vi "COMI WFM Start.vi"(5 "nMaxLoops":i32, 6 "nPPS":u32, 7 "nNumData":u32, 9 "pDataBuffer":sgl, 10 "ch":i32, 11 "hDevice":u32) -> (1 "pDataBuffer out":sgl, 2 "function return":i32, 3 "hDevice out":u32)   [LabVIEW 2017, in "Comidll.lvlib"]
doc: "long (COMI_WFM_Start) (HANDLE hDevice, int ch, float *pDataBuffer, \n unsigned int nNumData, unsigned int nPPS, int nMaxLoops);"
uses:
  <userlib>/Comidll/Comidll.lvlib
  <userlib>/Comidll/Comidll.dll
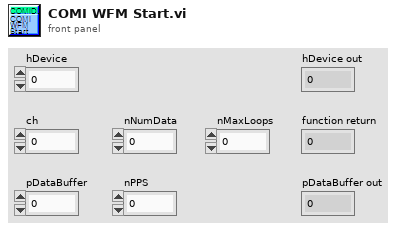
[diagram p1: front panel]
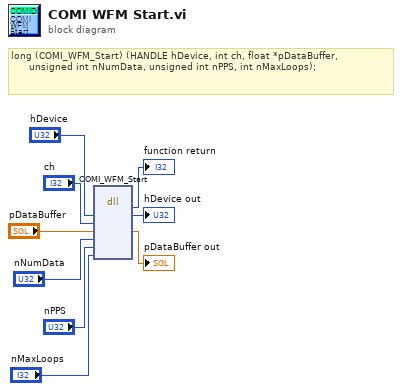
[diagram p0: block diagram]
diagram:
  # "long\t(COMI_WFM_Start) (HANDLE hDevice, int ch, float *pDataBuffer, \n\t\t\t\t\t\tunsigned int nNumData, unsigned int nPPS, int nMaxLoops);"
  n1 = dll-call lib="C:/Program Files/National Instruments/LabVIEW 2017/user.lib/Comidll/Comidll.*" fn="COMI_WFM_Start"("hDevice"="hDevice", "ch"="ch", "pDataBuffer"="pDataBuffer", "nNumData"="nNumData", "nPPS"="nPPS", "nMaxLoops"="nMaxLoops") -> (→"function return":i32, "hDevice"=→"hDevice out":u32, "pDataBuffer"=→"pDataBuffer out":sgl)  [unwired: 7 in, 2 out]
